vi "sub_frame_to_packets.vi"() -> ()   [LabVIEW 2014]
panel:
  out "packets":i16[][](array[numeric])
  in  "Cluster":cluster{i32, "Data String":string}
  in  "packet size":i32
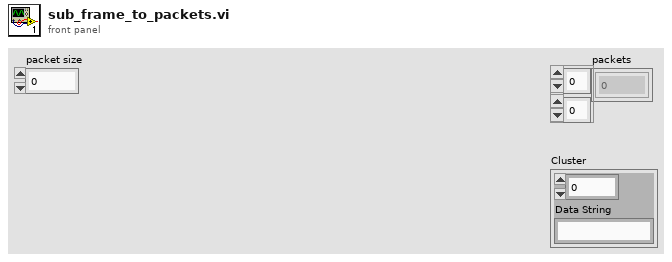
[diagram p1: front panel]
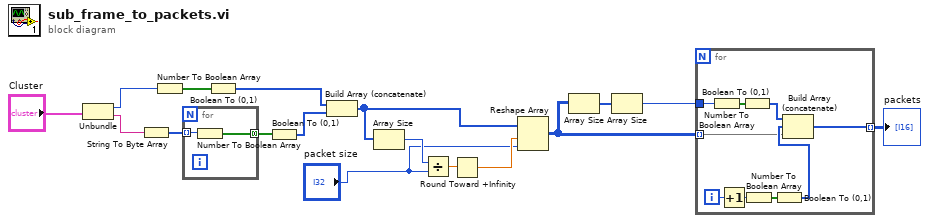
[diagram p0: block diagram]
diagram:
  n1 = Unbundle("Cluster") -> (w13:i32, "Data String"=w12:string)
  n2 = String To Byte Array(string=w12) -> (unsigned byte array=w16:u8[])
  n3 = Number To Boolean Array(number=w13) -> (Boolean array=w14:bool[])
  n4 = for {
    tunnel: w16 -> [w19] mode=indexing
    tunnel: [w18] -> w15 mode=concatenating
    n5 = Number To Boolean Array(number=w19) -> (Boolean array=w18:bool[])
  }
  n6 = Boolean To (0,1)(Boolean=w14) -> (0, 1=w10:i16[])
  n7 = Boolean To (0,1)(Boolean=w15) -> (0, 1=w11:i16[])
  n8 = Build Array (concatenate)(w10, w11) -> (w5:i16[])
  n9 = Array Size(array=w5) -> (size(s)=w9:i32)
  n10 = Divide(x=w9, y="packet size") -> (x/y=w8:dbl)
  n11 = Round Toward +Infinity(x=w8) -> (ceil(x): smallest int >= x=w7:dbl)
  n12 = Reshape Array(w5, w7, "packet size") -> (w4:i16[][])
  n13 = Array Size(array=w4) -> (size(s)=w2:i32[])
  n14 = Array Size(array=w2) -> (size(s)=w1:i32)
  n15 = for {
    tunnel: w4 -> [w25] mode=indexing
    tunnel: w1 -> [w23]
    tunnel: [w20] -> w3 mode=indexing
    i -> [w27]
    n16 = Number To Boolean Array(number=w23) -> (Boolean array=w24:bool[])
    n17 = Increment(x=w27) -> (x+1=w21:i32)
    n18 = Boolean To (0,1)(Boolean=w24) -> (0, 1=w22:i16[])
    n19 = Number To Boolean Array(number=w21) -> (Boolean array=w28:bool[])
    n20 = Boolean To (0,1)(Boolean=w28) -> (0, 1=w26:i16[])
    n21 = Build Array (concatenate)(w22, w26, w25) -> (w20:i16[])
  }
  "packets" <- w3
